vi "In_S10F2.vi"(8 "error in (no error)":errorcluster, 11 "S10 Message Class in":refnum<class "S10 Message Class.lvclass">) -> (0 "error out":errorcluster, 1 "OK?":bool, 2 "S10F2":T1, 3 "S10 Message Class out":refnum<class "S10 Message Class.lvclass">)   [LabVIEW 2020, in "SECS Communication.lvlib" / "S10 Message Class.lvclass"]
uses:
  S10 Message Class.lvclass
  D:/Dropbox/SECS/SECS_GEM v1.0.6/Com/SECS Communication/SECS-II Class/SECS-II Class.lvclass
  S10F2.ctl
  SECS-II Class/SECS-II Class.lvclass/SECS-II Class.ctl
  SECS-II Class/Variant To Data_Binary.vi
  SECS-II Class/SECS-II Class.lvclass
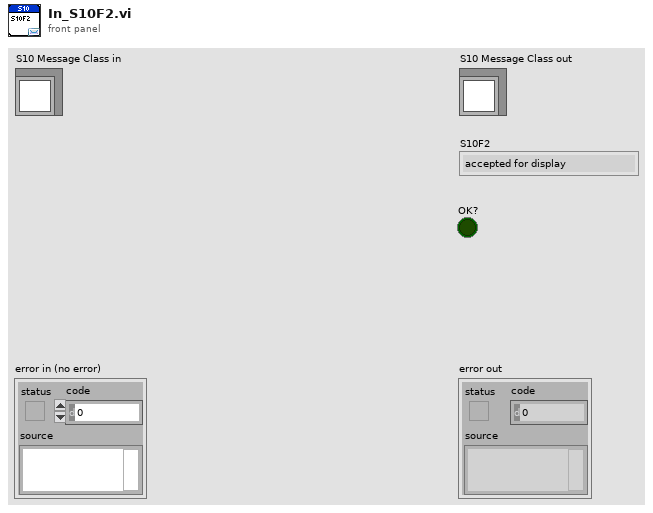
[diagram p1: front panel]
types:
  T1 = typedef "SECS Communication.lvlib/S10 Message Class.lvclass/S10F2.ctl" = enum8{"accepted for display", "message will not be displayed", "terminal not available"}
  T2 = typedef "SECS Communication.lvlib/SECS-II Class.lvclass/Message Data.ctl" = cluster{"Index":i32, "Data Item Format":T3, "Format Code":T4, "Parent Index":i32, "Child Index":i32[], "Data":variant}
  T3 = typedef "SECS Communication.lvlib/SECS-II Class.lvclass/Data Item Format.ctl" = enum16{"Data Type", "Value"}
  T4 = typedef "SECS Communication.lvlib/SECS-II Class.lvclass/Format Code.ctl" = enum16{"L", "A", "B", "Boolean", "J", "I1", "I2", "I4", "I8", "U1", "U2", "U4", "U8", "F4", "F8", "Char"}
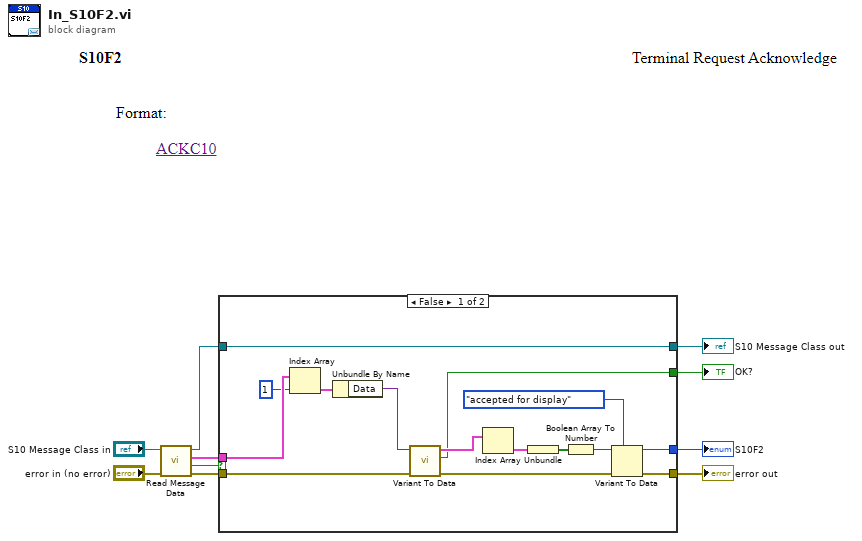
[diagram p0: block diagram]
diagram:
  n1 = call "Read Message Data.vi"("error in (no error)"="error in (no error)", "SECS-II Class in"="S10 Message Class in") -> ("error out"=w10:errorcluster, "Empty?"=w4:bool, "Message Data"=w9:T2[], "SECS-II Class out"=w2:refnum<class "S10 Message Class.lvclass">)  [unwired: 6 in]
  n2 = case shown="False" w4 {
    tunnel: w10 -> [w23 w27]
    tunnel: w9 -> [w22 _]
    tunnel: [w14 w27] -> w8
    tunnel: [w13 _] -> w7
    tunnel: [w12 w26] -> w3
    tunnel: w2 -> [w12 w26]
    tunnel: [w11 _] -> w1
    frame False {
      n3 = Index Array(array=w22, index=1) -> (element=w24:T2)
      n4 = Unbundle By Name(w24) -> ("Data"=w25:variant)
      n5 = call-poly "Variant To Data.vi"("error in (no error)"=w23, "Variant"=w25) -> ("error out"=w17:errorcluster, "OK?"=w11:bool, "Data Cluster"=w20:cluster{"Data":bool[]}[])  [unwired: 7 in]
      n6 = Index Array(array=w20) -> (element=w18:cluster{"Data":bool[]})  [unwired: 1 in]
      n7 = Unbundle(w18) -> ("Data"=w19:bool[])
      n8 = Boolean Array To Number(Boolean array=w19) -> (number=w16:u32)
      n9 = Variant To Data(error in=w17, type=S10F2."accepted for display" ("S10F2"), Variant=w16) -> (data=w13:T1, error out=w14:errorcluster)
    }
    frame True {
    }
  }
  "error out" <- w8
  "S10 Message Class out" <- w3
  "S10F2" <- w7
  "OK?" <- w1
